vi "1.vi"() -> ()   [LabVIEW 2011]
uses:
  <vilib>/Instr/_visa.llb/VISA Configure Serial Port (Instr).vi
panel:
  in  "停止位":u16(ring)=10 items=["1.0"=10, "1.5"=15, "2.0"=20]
  in  "校验位":enum16{"None", "Odd", "Even", "Mark", "Space"}(ring)=enum."Even"
  in  "数据位":u16=7
  in  "波特率":u32=9600
  in  "串口号":refnum<visa-resource-name>="COM3"
  in  "D7 2":u16
  in  "D3 2":u16
  in  "D1 2":u16
  in  "D2 2":u16
  in  "D0 2":u16
  in  "D5 2":u16
  in  "D6 2":u16
  in  "D4 2":u16
  in  "D9 2":u16
  in  "D8 2":u16
  in  "M31 2":bool
  in  "M30 2":bool
  in  "M29 2":bool
  in  "M28 2":bool
  in  "M27 2":bool
  in  "M26 2":bool
  in  "M25 2":bool
  in  "M24 2":bool
  in  "M23 2":bool
  in  "M22 2":bool
  in  "M21 2":bool
  in  "M20 2":bool
  in  "M19 2":bool
  in  "M18 2":bool
  in  "M17 2":bool
  in  "M16 2":bool
  in  "M15 2":bool
  in  "M14 2":bool
  in  "M13 2":bool
  in  "M12 2":bool
  in  "M11 2":bool
  in  "M10 2":bool
  in  "M9 2":bool
  in  "M7 2":bool
  in  "M8 2":bool
  in  "M6 2":bool
  in  "M5 2":bool
  in  "M4 2":bool
  in  "M3 2":bool
  in  "M2 2":bool
  in  "M1 2":bool
  in  "M0 2":bool
  in  "Y17 2":bool
  in  "Y16 2":bool
  in  "Y15 2":bool
  in  "Y14 2":bool
  in  "Y13 2":bool
  in  "Y12 2":bool
  in  "Y11 2":bool
  in  "Y10 2":bool
  in  "Y7 2":bool
  in  "Y6 2":bool
  in  "Y5 2":bool
  in  "Y4 2":bool
  in  "Y3 2":bool
  in  "Y2 2":bool
  in  "Y1 2":bool
  in  "Y0 2":bool
  in  "Y35 2":bool
  in  "Y37 2":bool
  in  "Y36 2":bool
  in  "Y34 2":bool
  in  "Y33 2":bool
  in  "Y32 2":bool
  in  "Y31 2":bool
  in  "Y30 2":bool
  in  "Y27 2":bool
  in  "Y26 2":bool
  in  "Y25 2":bool
  in  "Y24 2":bool
  in  "Y23 2":bool
  in  "Y22 2":bool
  in  "Y21 2":bool
  in  "Y20 2":bool
  out "X17":bool
  out "X16":bool
  out "D0":i32
  out "D1":i32
  out "D2":i32
  out "D3":i32
  out "D7":i32
  out "D6":i32
  out "D5":i32
  out "D4":i32
  out "D9":i32
  out "D8":i32
  out "Y37":bool
  out "Y36":bool
  out "Y35":bool
  out "Y34":bool
  out "Y33":bool
  out "Y32":bool
  out "Y31":bool
  out "Y30":bool
  out "Y27":bool
  out "Y26":bool
  out "Y25":bool
  out "Y24":bool
  out "Y23":bool
  out "Y22":bool
  out "Y21":bool
  out "Y20":bool
  out "Y17":bool
  out "Y16":bool
  out "Y15":bool
  out "Y14":bool
  out "Y13":bool
  out "Y12":bool
  out "Y11":bool
  out "Y10":bool
  out "Y7":bool
  out "Y6":bool
  out "Y5":bool
  out "Y4":bool
  out "Y3":bool
  out "Y2":bool
  out "Y1":bool
  out "Y0":bool
  out "M31":bool
  out "M30":bool
  out "M29":bool
  out "M28":bool
  out "M27":bool
  out "M26":bool
  out "M25":bool
  out "M24":bool
  out "M23":bool
  out "M22":bool
  out "?":bool
  out "M20":bool
  out "M19":bool
  out "M18":bool
  out "M17":bool
  out "M16":bool
  out "M15":bool
  out "M14":bool
  out "M13":bool
  out "M12":bool
  out "M11":bool
  out "M10":bool
  out "M9":bool
  out "M8":bool
  out "M7":bool
  out "M6":bool
  out "M5":bool
  out "M4":bool
  out "M3":bool
  out "M2":bool
  out "M1":bool
  out "M0":bool
  out "X37":bool
  out "X36":bool
  out "X35":bool
  out "X34":bool
  out "X33":bool
  out "X32":bool
  out "X31":bool
  out "X30":bool
  out "X27":bool
  out "X26":bool
  out "X25":bool
  out "X24":bool
  out "X23":bool
  out "X22":bool
  out "X21":bool
  out "X20":bool
  out "X15":bool
  out "X14":bool
  out "X13":bool
  out "X12":bool
  out "X11":bool
  out "X10":bool
  out "X7":bool
  out "X6":bool
  out "X5":bool
  out "X4":bool
  out "X3":bool
  out "X2":bool
  out "X1":bool
  out "X0":bool
  in  "停止":bool
  # "LabVIEW和三菱FX系列PLC编程口通讯源码"
  # "读Y0-Y7"
  # "读X0-MX7"
  # "读M0-M7"
  # "读Y10-Y17"
  # "读M10-M17"
  # "读X10-X17"
  # "写Y20-Y27"
  # "读M20-M27"
  # "读X20-X27"
  # "读M30-M37"
  # "写Y30-Y37"
  # "读X30-X37"
  # "写Y0-Y7"
  # "写M0-M7"
  # "写D0-D4"
  # "写Y10-Y17"
  # "写M10-M17"
  # "写D5-D9"
  # "写Y20-Y27"
  # "写M20-M27"
  # "读D0-D4"
  # "写Y30-Y37"
  # "写M30-M37"
  # "读D5-D9"
  # "确保程序运行正常 设置好串口号 . 波特率.  然后再启动程序"
  # "有需要源码的请联系.张杰伟 18368748504"
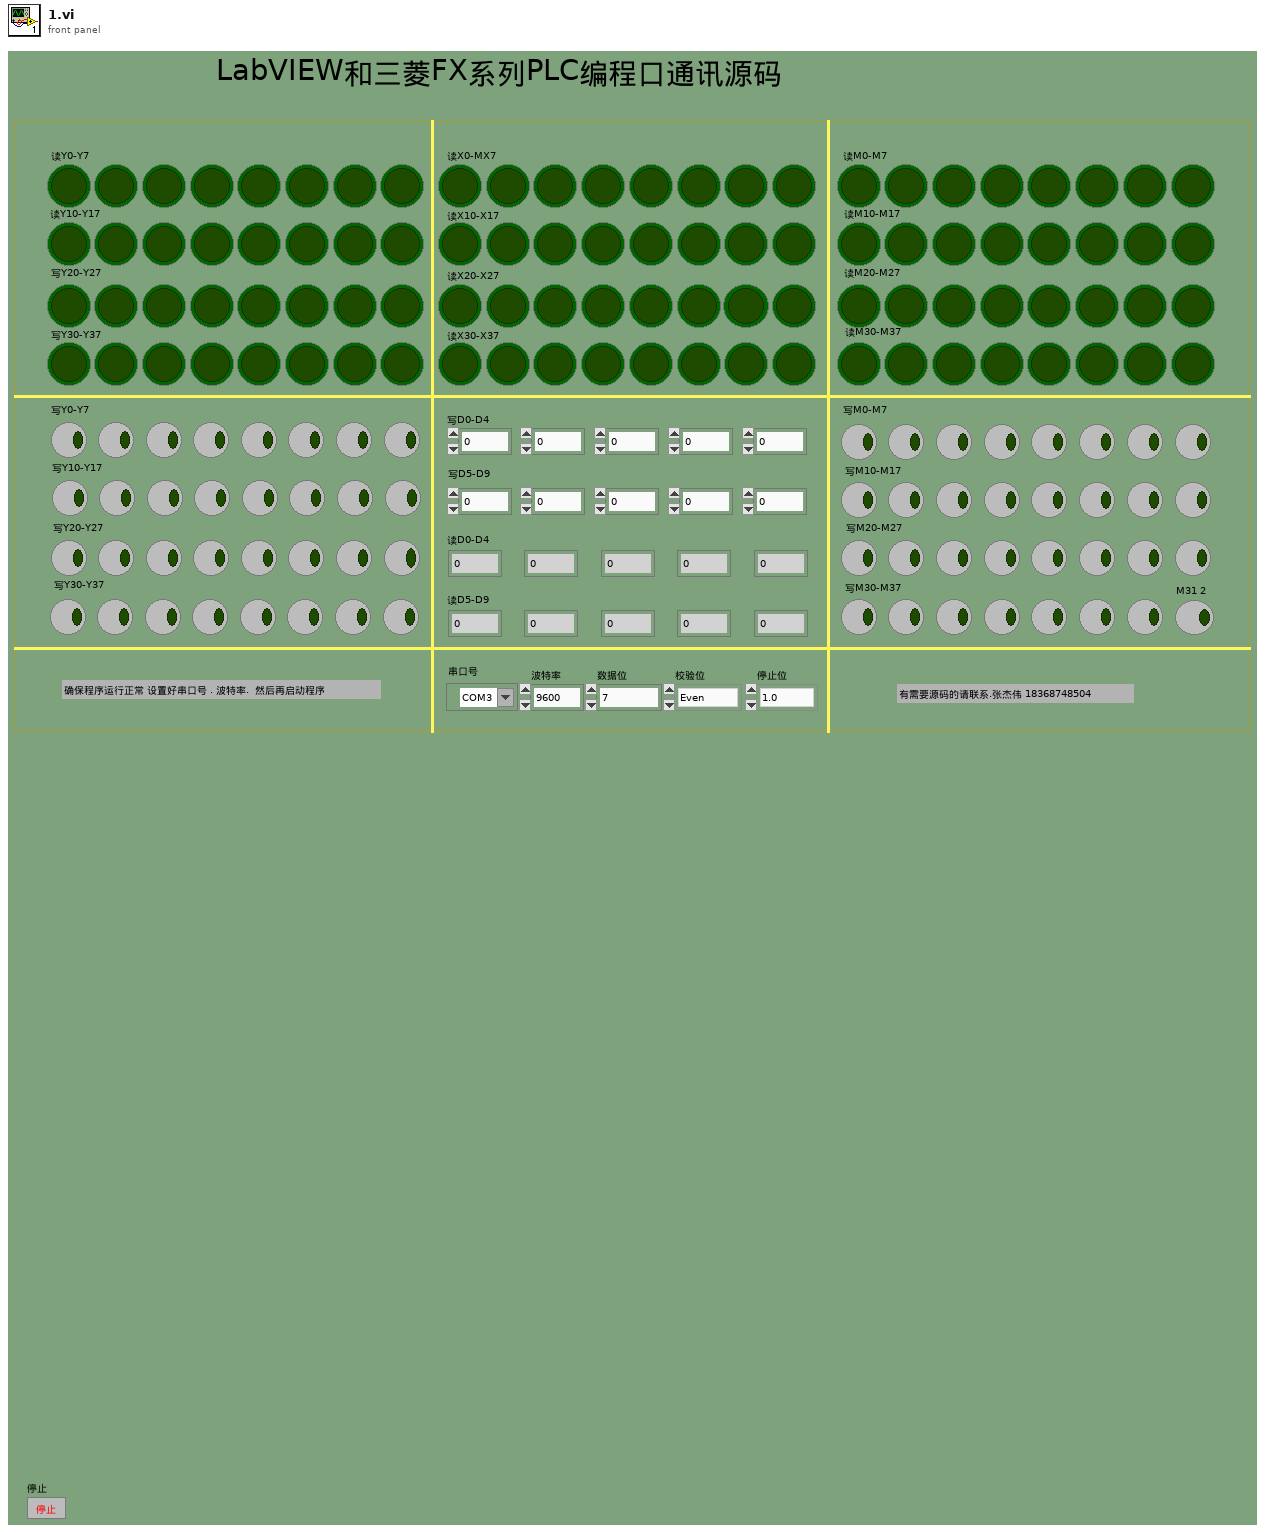
[diagram p1: front panel]
types:
  T1 = cluster{"D0":u16, "D1":u16, "D3":u16, "D2":u16, "D5":u16, "D4":u16, "D7":u16, "D6":u16, "D9":u16, "D8":u16}
  T2 = cluster{"M16":bool, "M17":bool, "M18":bool, "M19":bool, "M20":bool, "M21":bool, "M22":bool, "M23":bool, "M24":bool, "M25":bool, "M26":bool, "M27":bool, "M28":bool, "M29":bool, "M30":bool, "M31":bool}
  T3 = cluster{"M0":bool, "M1":bool, "M2":bool, "M3":bool, "M4":bool, "M5":bool, "M6":bool, "M7":bool, "M8":bool, "M9":bool, "M10":bool, "M11":bool, "M12":bool, "M13":bool, "M14":bool, "M15":bool}
  T4 = cluster{"Y0":bool, "Y1":bool, "Y2":bool, "Y3":bool, "Y4":bool, "Y5":bool, "Y6":bool, "Y7":bool, "Y10":bool, "Y11":bool, "Y12":bool, "Y13":bool, "Y14":bool, "Y15":bool, "Y16":bool, "Y17":bool}
  T5 = cluster{"Y20":bool, "Y21":bool, "Y22":bool, "Y23":bool, "Y24":bool, "Y25":bool, "Y26":bool, "Y27":bool, "Y30":bool, "Y31":bool, "Y32":bool, "Y33":bool, "Y34":bool, "Y35":bool, "Y36":bool, "Y37":bool}
  T6 = cluster{"X0":bool, "X1":bool, "X2":bool, "X3":bool, "X4":bool, "X5":bool, "X6":bool, "X7":bool, "X10":bool, "X11":bool, "X12":bool, "X13":bool, "X14":bool, "X15":bool, "X16":bool, "X17":bool}
  T7 = cluster{"X20":bool, "X21":bool, "X22":bool, "X23":bool, "X24":bool, "X25":bool, "X26":bool, "X27":bool, "X30":bool, "X31":bool, "X32":bool, "X33":bool, "X34":bool, "X35":bool, "X36":bool, "X37":bool}
  T8 = cluster{"D0":i32, "D1":i32, "D2":i32, "D3":i32, "D4":i32, "D5":i32, "D6":i32, "D7":i32, "D8":i32, "D9":i32}
  T9 = cluster{"D0":bool, "D1":bool, "D3":bool, "D2":bool, "D5":bool, "D4":bool, "D7":bool, "D6":bool, "D9":bool, "D8":bool}
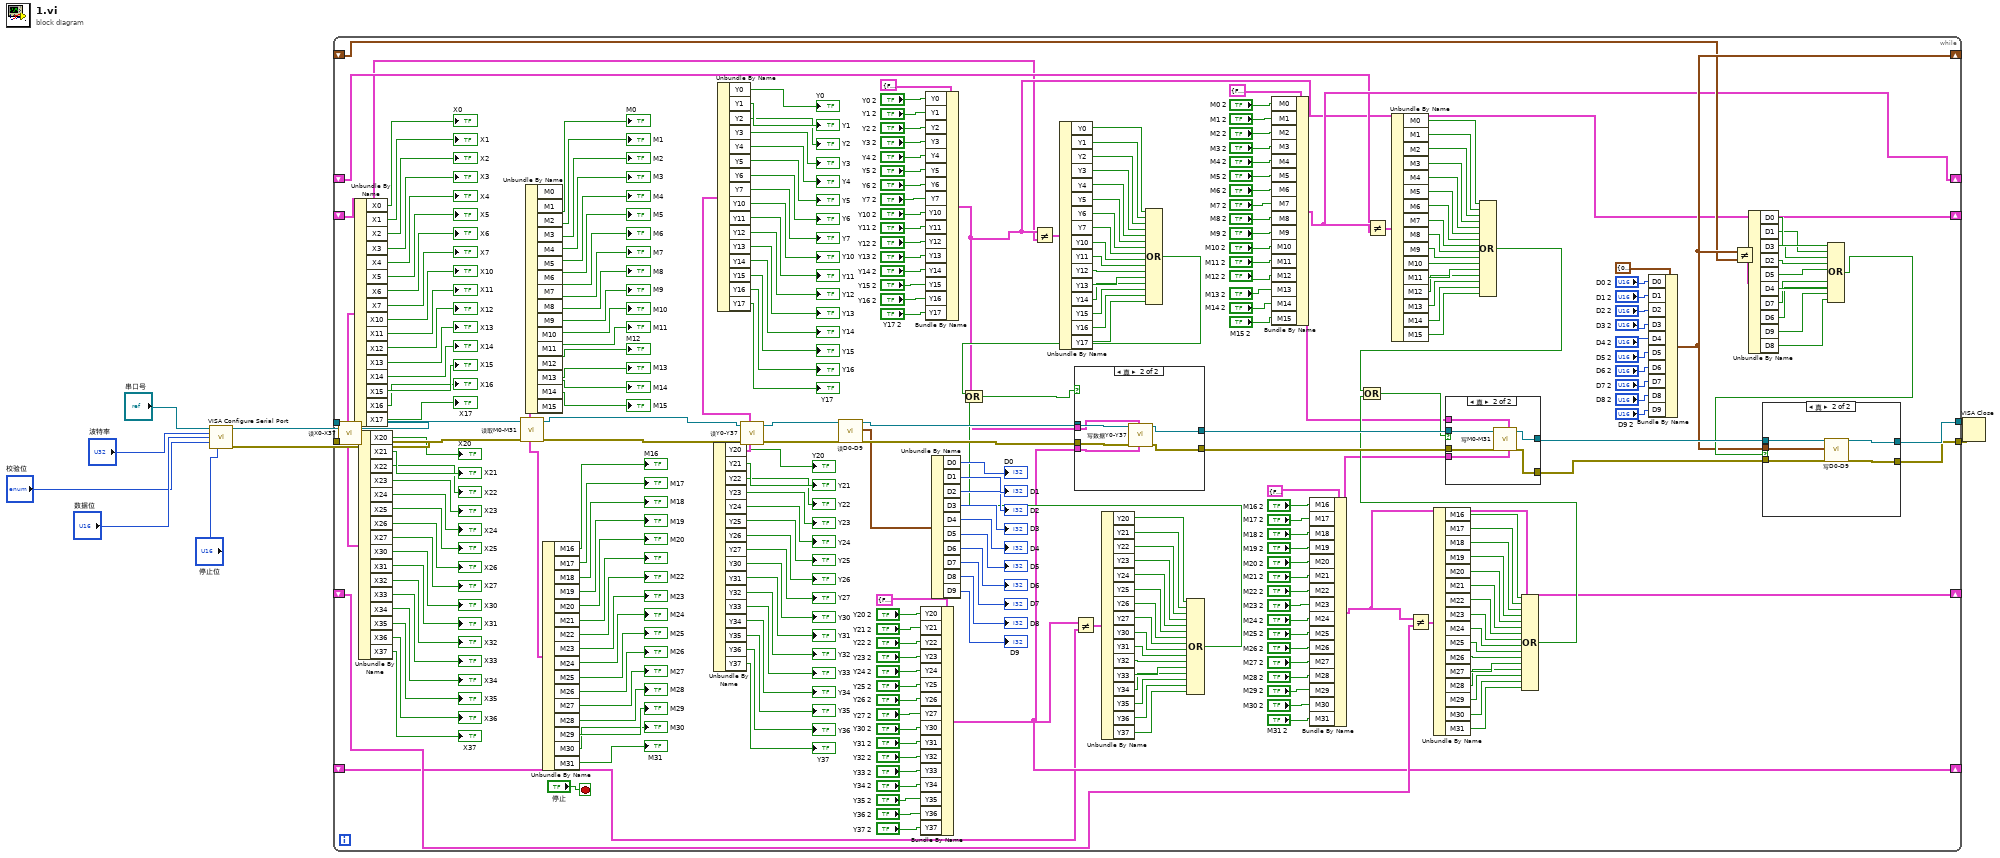
[diagram p0: block diagram]
diagram:
  n1 = call-poly "VISA Configure Serial Port"("VISA resource name"="串口号", "baud rate (9600)"="波特率", "data bits (8)"="数据位", "parity (0:none)"="校验位", "stop bits (10: 1 bit)"="停止位") -> ("VISA resource name out"=w9:refnum<visa-resource-name>, "error out"=w8:errorcluster)  [unwired: 9 in]
  n2 = while {
    tunnel: w9 -> [w313]
    tunnel: w8 -> [w312]
    tunnel: [w197] -> w2
    tunnel: [w196] -> w1
    shift-right: [w87] -> _
    shift-left: _ -> [w86]
    shift-right: [w85] -> _
    shift-left: _ -> [w67]
    shift-right: [w49] -> _
    shift-left: _ -> [w48]
    shift-right: [w30] -> _
    shift-left: _ -> [w29]
    shift-right: [w28] -> _
    shift-left: _ -> [w10]
    stop <- "停止" stop-if-true
    n3 = call "读X0-X37.vi"("VISA资源名称"=w313, "错误输入（无错误）"=w312) -> ("X0-X17"=w305:T6, "X20-X37"=w304:T7, "VISA资源名称输出"=w311:refnum<visa-resource-name>, "错误输出"=w310:errorcluster)  [unwired: 4 in]
    n4 = Unbundle By Name(w305) -> ("X0"=→"X0":bool, "X1"=→"X1":bool, "X2"=→"X2":bool, "X3"=→"X3":bool, "X4"=→"X4":bool, "X5"=→"X5":bool, "X6"=→"X6":bool, "X7"=→"X7":bool, "X10"=→"X10":bool, "X11"=→"X11":bool, "X12"=→"X12":bool, "X13"=→"X13":bool, "X14"=→"X14":bool, "X15"=→"X15":bool, "X16"=→"X16":bool, "X17"=→"X17":bool)
    n5 = Unbundle By Name(w304) -> ("X20"=→"X20":bool, "X21"=→"X21":bool, "X22"=→"X22":bool, "X23"=→"X23":bool, "X24"=→"X24":bool, "X25"=→"X25":bool, "X26"=→"X26":bool, "X27"=→"X27":bool, "X30"=→"X30":bool, "X31"=→"X31":bool, "X32"=→"X32":bool, "X33"=→"X33":bool, "X34"=→"X34":bool, "X35"=→"X35":bool, "X36"=→"X36":bool, "X37"=→"X37":bool)
    n6 = call "读取M0-M31.vi"("错误输入（无错误）"=w310, "VISA资源名称"=w311) -> ("错误输出"=w308:errorcluster, "VISA资源名称输出"=w309:refnum<visa-resource-name>, "M16-M21"=w272:T2, "M0-M15"=w273:T3)  [unwired: 6 in]
    n7 = Unbundle By Name(w273) -> ("M0"=→"M0":bool, "M1"=→"M1":bool, "M2"=→"M2":bool, "M3"=→"M3":bool, "M4"=→"M4":bool, "M5"=→"M5":bool, "M6"=→"M6":bool, "M7"=→"M7":bool, "M8"=→"M8":bool, "M9"=→"M9":bool, "M10"=→"M10":bool, "M11"=→"M11":bool, "M12"=→"M12":bool, "M13"=→"M13":bool, "M14"=→"M14":bool, "M15"=→"M15":bool)
    n8 = Unbundle By Name(w272) -> ("M16"=→"M16":bool, "M17"=→"M17":bool, "M18"=→"M18":bool, "M19"=→"M19":bool, "M20"=→"M20":bool, "M21"=→"?":bool, "M22"=→"M22":bool, "M23"=→"M23":bool, "M24"=→"M24":bool, "M25"=→"M25":bool, "M26"=→"M26":bool, "M27"=→"M27":bool, "M28"=→"M28":bool, "M29"=→"M29":bool, "M30"=→"M30":bool, "M31"=→"M31":bool)
    n9 = call "读Y0-Y37.vi"("VISA资源名称"=w309, "错误输入（无错误）"=w308) -> ("Y0-Y17"=w239:T4, "Y20-Y37"=w238:T5, "VISA资源名称输出"=w307:refnum<visa-resource-name>, "错误输出"=w306:errorcluster)  [unwired: 4 in]
    n10 = Unbundle By Name(w238) -> ("Y20"=→"Y20":bool, "Y21"=→"Y21":bool, "Y22"=→"Y22":bool, "Y23"=→"Y23":bool, "Y24"=→"Y24":bool, "Y25"=→"Y25":bool, "Y26"=→"Y26":bool, "Y27"=→"Y27":bool, "Y30"=→"Y30":bool, "Y31"=→"Y31":bool, "Y32"=→"Y32":bool, "Y33"=→"Y33":bool, "Y34"=→"Y34":bool, "Y35"=→"Y35":bool, "Y36"=→"Y36":bool, "Y37"=→"Y37":bool)
    n11 = Unbundle By Name(w239) -> ("Y0"=→"Y0":bool, "Y1"=→"Y1":bool, "Y2"=→"Y2":bool, "Y3"=→"Y3":bool, "Y4"=→"Y4":bool, "Y5"=→"Y5":bool, "Y6"=→"Y6":bool, "Y7"=→"Y7":bool, "Y10"=→"Y10":bool, "Y11"=→"Y11":bool, "Y12"=→"Y12":bool, "Y13"=→"Y13":bool, "Y14"=→"Y14":bool, "Y15"=→"Y15":bool, "Y16"=→"Y16":bool, "Y17"=→"Y17":bool)
    n12 = call "读D0-D9.vi"("VISA资源名称"=w307, "错误输入（无错误）"=w306) -> ("VISA资源名称输出"=w203:refnum<visa-resource-name>, "D0-D9"=w116:T8, "错误输出"=w202:errorcluster)  [unwired: 15 in]
    n13 = Bundle By Name(cluster=T5 {"Y20"=FALSE, "Y21"=FALSE, "Y22"=FALSE, "Y23"=FALSE, "Y24"=FALSE, "Y25"=FALSE, "Y26"=FALSE, "Y27"=FALSE, "Y30"=FALSE, "Y31"=FALSE, "Y32"=FALSE, "Y33"=FALSE, "Y34"=FALSE, "Y35"=FALSE, "Y36"=FALSE, "Y37"=FALSE} ("Y20-Y37"), "Y20"="Y20 2", "Y21"="Y21 2", "Y22"="Y22 2", "Y23"="Y23 2", "Y24"="Y24 2", "Y25"="Y25 2", "Y26"="Y26 2", "Y27"="Y27 2", "Y30"="Y30 2", "Y31"="Y31 2", "Y32"="Y32 2", "Y33"="Y33 2", "Y34"="Y34 2", "Y35"="Y35 2", "Y36"="Y36 2", "Y37"="Y37 2") -> (w28:T5)
    n14 = Bundle By Name ("按名称捆绑")(cluster=T4 {"Y0"=FALSE, "Y1"=FALSE, "Y2"=FALSE, "Y3"=FALSE, "Y4"=FALSE, "Y5"=FALSE, "Y6"=FALSE, "Y7"=FALSE, "Y10"=FALSE, "Y11"=FALSE, "Y12"=FALSE, "Y13"=FALSE, "Y14"=FALSE, "Y15"=FALSE, "Y16"=FALSE, "Y17"=FALSE} ("Y0-Y17"), "Y0"="Y0 2", "Y1"="Y1 2", "Y2"="Y2 2", "Y3"="Y3 2", "Y4"="Y4 2", "Y5"="Y5 2", "Y6"="Y6 2", "Y7"="Y7 2", "Y10"="Y10 2", "Y11"="Y11 2", "Y12"="Y12 2", "Y13"="Y13 2", "Y14"="Y14 2", "Y15"="Y15 2", "Y16"="Y16 2", "Y17"="Y17 2") -> (w49:T4)
    n15 = Unbundle By Name(w116) -> ("D0"=→"D0":i32, "D1"=→"D1":i32, "D2"=→"D2":i32, "D3"=→"D3":i32, "D4"=→"D4":i32, "D5"=→"D5":i32, "D6"=→"D6":i32, "D7"=→"D7":i32, "D8"=→"D8":i32, "D9"=→"D9":i32)
    n16 = Not Equal?(x=w49, y=w48) -> (x != y?=w66:T4)
    n17 = Unbundle By Name(w66) -> ("Y0"=w65:bool, "Y1"=w64:bool, "Y2"=w63:bool, "Y3"=w62:bool, "Y4"=w61:bool, "Y5"=w60:bool, "Y6"=w59:bool, "Y7"=w58:bool, "Y10"=w57:bool, "Y11"=w56:bool, "Y12"=w55:bool, "Y13"=w54:bool, "Y14"=w53:bool, "Y15"=w52:bool, "Y16"=w51:bool, "Y17"=w50:bool)
    n18 = Not Equal?(x=w28, y=w10) -> (x != y?=w27:T5)
    n19 = Unbundle By Name(w27) -> ("Y20"=w26:bool, "Y21"=w25:bool, "Y22"=w24:bool, "Y23"=w23:bool, "Y24"=w22:bool, "Y25"=w21:bool, "Y26"=w20:bool, "Y27"=w19:bool, "Y30"=w18:bool, "Y31"=w17:bool, "Y32"=w16:bool, "Y33"=w15:bool, "Y34"=w14:bool, "Y35"=w13:bool, "Y36"=w12:bool, "Y37"=w11:bool)
    n20 = Compound Arithmetic op=OR(w65, w64, w63, w62, w61, w60, w59, w58, w57, w56, w55, w54, w53, w52, w51, w50) -> (w99:bool)
    n21 = Compound Arithmetic op=OR(w26, w25, w24, w23, w22, w21, w20, w19, w18, w17, w16, w15, w14, w13, w12, w11) -> (w101:bool)
    n22 = Compound Arithmetic op=OR(w99, w101) -> (w100:bool)
    n23 = case shown="真" w100 {
      tunnel: w203 -> [w315 w322]
      tunnel: w202 -> [w316 w321]
      tunnel: [w315 w320] -> w201
      tunnel: [w316 w319] -> w200
      tunnel: w49 -> [_ w318]
      tunnel: w28 -> [_ w317]
      frame False {
      }
      frame True {
        n24 = call "写数据Y0-Y37.vi"("Y20-Y37"=w317, "Y0-Y17"=w318, "错误输入（无错误）"=w321, "VISA资源名称"=w322) -> ("错误输出"=w319:errorcluster, "VISA资源名称输出"=w320:refnum<visa-resource-name>)  [unwired: 6 in]
      }
    }
    n25 = Bundle By Name(cluster=T3 {"M0"=FALSE, "M1"=FALSE, "M2"=FALSE, "M3"=FALSE, "M4"=FALSE, "M5"=FALSE, "M6"=FALSE, "M7"=FALSE, "M8"=FALSE, "M9"=FALSE, "M10"=FALSE, "M11"=FALSE, "M12"=FALSE, "M13"=FALSE, "M14"=FALSE, "M15"=FALSE} ("M0-M15"), "M0"="M0 2", "M1"="M1 2", "M2"="M2 2", "M3"="M3 2", "M4"="M4 2", "M5"="M5 2", "M6"="M6 2", "M7"="M7 2", "M8"="M8 2", "M9"="M9 2", "M10"="M10 2", "M11"="M11 2", "M12"="M12 2", "M13"="M13 2", "M14"="M14 2", "M15"="M15 2") -> (w85:T3)
    n26 = Bundle By Name(cluster=T2 {"M16"=FALSE, "M17"=FALSE, "M18"=FALSE, "M19"=FALSE, "M20"=FALSE, "M21"=FALSE, "M22"=FALSE, "M23"=FALSE, "M24"=FALSE, "M25"=FALSE, "M26"=FALSE, "M27"=FALSE, "M28"=FALSE, "M29"=FALSE, "M30"=FALSE, "M31"=FALSE} ("M16-M31"), "M16"="M16 2", "M17"="M17 2", "M18"="M18 2", "M19"="M19 2", "M20"="M20 2", "M21"="M21 2", "M22"="M22 2", "M23"="M23 2", "M24"="M24 2", "M25"="M25 2", "M26"="M26 2", "M27"="M27 2", "M28"="M28 2", "M29"="M29 2", "M30"="M30 2", "M31"="M31 2") -> (w30:T2)
    n27 = Not Equal?(x=w85, y=w67) -> (x != y?=w84:T3)
    n28 = Unbundle By Name(w84) -> ("M0"=w83:bool, "M1"=w82:bool, "M2"=w81:bool, "M3"=w80:bool, "M4"=w79:bool, "M5"=w78:bool, "M6"=w77:bool, "M7"=w76:bool, "M8"=w75:bool, "M9"=w74:bool, "M10"=w73:bool, "M11"=w72:bool, "M12"=w71:bool, "M13"=w70:bool, "M14"=w69:bool, "M15"=w68:bool)
    n29 = Not Equal?(x=w30, y=w29) -> (x != y?=w47:T2)
    n30 = Unbundle By Name(w47) -> ("M16"=w46:bool, "M17"=w45:bool, "M18"=w44:bool, "M19"=w43:bool, "M20"=w42:bool, "M21"=w41:bool, "M22"=w40:bool, "M23"=w39:bool, "M24"=w38:bool, "M25"=w37:bool, "M26"=w36:bool, "M27"=w35:bool, "M28"=w34:bool, "M29"=w33:bool, "M30"=w32:bool, "M31"=w31:bool)
    n31 = Compound Arithmetic op=OR(w83, w82, w81, w80, w79, w78, w77, w76, w75, w74, w73, w72, w71, w70, w69, w68) -> (w104:bool)
    n32 = Compound Arithmetic op=OR(w46, w45, w44, w43, w42, w41, w40, w39, w38, w37, w36, w35, w34, w33, w32, w31) -> (w103:bool)
    n33 = Compound Arithmetic op=OR(w104, w103) -> (w102:bool)
    n34 = case shown="真" w102 {
      tunnel: w201 -> [w324 w330]
      tunnel: w200 -> [w323 w329]
      tunnel: [w324 w328] -> w199
      tunnel: [w323 w327] -> w198
      tunnel: w85 -> [_ w326]
      tunnel: w30 -> [_ w325]
      frame False {
      }
      frame True {
        n35 = call "写M0-M31.vi"("M16-M31"=w325, "M0-M15"=w326, "错误输入（无错误）"=w329, "VISA资源名称"=w330) -> ("错误输出"=w327:errorcluster, "VISA资源名称输出"=w328:refnum<visa-resource-name>)  [unwired: 6 in]
      }
    }
    n36 = Bundle By Name(cluster=T1 {"D0"=0, "D1"=0, "D3"=0, "D2"=0, "D5"=0, "D4"=0, "D7"=0, "D6"=0, "D9"=0, "D8"=0} ("簇"), "D0"="D0 2", "D1"="D1 2", "D2"="D2 2", "D3"="D3 2", "D4"="D4 2", "D5"="D5 2", "D6"="D6 2", "D7"="D7 2", "D8"="D8 2", "D9"="D9 2") -> (w87:T1)
    n37 = Not Equal?(x=w87, y=w86) -> (x != y?=w98:T9)
    n38 = Unbundle By Name(w98) -> ("D0"=w97:bool, "D1"=w96:bool, "D3"=w95:bool, "D2"=w94:bool, "D5"=w93:bool, "D4"=w92:bool, "D7"=w91:bool, "D6"=w90:bool, "D9"=w89:bool, "D8"=w88:bool)
    n39 = Compound Arithmetic op=OR(w97, w96, w95, w94, w93, w92, w91, w90, w89, w88) -> (w105:bool)
    n40 = case shown="真" w105 {
      tunnel: w199 -> [w332 w337]
      tunnel: w198 -> [w331 w336]
      tunnel: [w332 w335] -> w197
      tunnel: [w331 w334] -> w196
      tunnel: w87 -> [_ w333]
      frame False {
      }
      frame True {
        n41 = call "写D0-D9.vi"("VISA资源名称"=w337, "簇"=w333, "错误输入（无错误）"=w336) -> ("VISA资源名称输出"=w335:refnum<visa-resource-name>, "错误输出"=w334:errorcluster)  [unwired: 15 in]
      }
    }
  }
  n42 = VISA Close(VISA resource name=w2, error in (no error)=w1) -> ()  [unwired: 1 out]
